vi "Set File Node.vi"(6 "Path":path, 7 "Extension":string, 8 "error in (no error)":errorcluster, 9 "Name":string, 10 "guid":string="3a41ca74-36ec-4aff-9219-9d05c8f91208", 11 "Doc in":refnum<k24>) -> (0 "error out":errorcluster, 3 "Doc out":refnum<k24>)   [LabVIEW 2013, in "Project Wizard.lvlib"]
uses:
  NationalInstruments.VeriStand.SystemStorage
  Project Wizard.lvlib
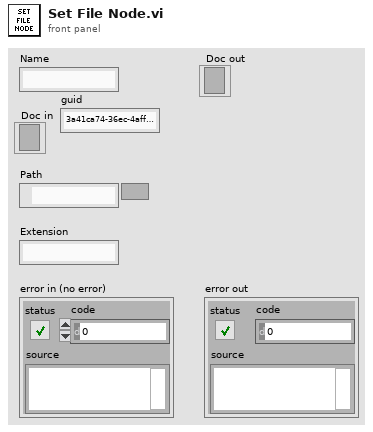
[diagram p1: front panel]
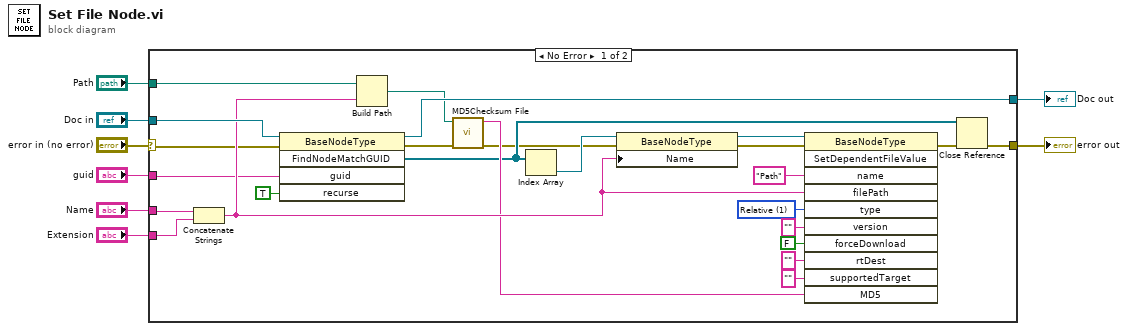
[diagram p0: block diagram]
diagram:
  n1 = case shown="No Error" "error in (no error)" {
    selector: "error in (no error)" -> [w12 w35]
    tunnel: "Doc in" -> [w33 w34]
    tunnel: "Name" -> [w32 _]
    tunnel: "Path" -> [w31 _]
    tunnel: [w29 w34] -> w5
    tunnel: [w28 w35] -> w4
    tunnel: "Extension" -> [w21 _]
    tunnel: "guid" -> [w11 _]
    frame No Error {
      w20 = 1 items=["Absolute", "Relative", "ToCommonDocDir", "ToApplicationDataDir"] ("type")
      n2 = Concatenate Strings(w32, w21) -> (w30:string)
      n3 = invoke class="BaseNodeType" method="FindNodeMatchGUID"(reference=w33, error in=w12, "guid"=w11, "recurse"=TRUE) -> (reference out=w29:refnum<k24>, error out=w10:errorcluster, "FindNodeMatchGUID"=w13:refnum<k24>[])  [unwired: 1 in, 2 out]
      n4 = Build Path(base path=w31, name or relative path=w30) -> (appended path=w27:path)
      n5 = call <vilib>:"MD5Checksum File.vi"("error in (no error)"=w10, "Path"=w27) -> ("error out"=w9:errorcluster, "MD5 message-digest"=w22:string)  [unwired: 8 in]
      n6 = Index Array(array=w13) -> (element=w18:refnum<k24>)  [unwired: 1 in]
      n7 = property class="BaseNodeType"(reference=w18, error in=w9, "Name"=w30) -> (reference out=w17:refnum<k24>, error out=w16:errorcluster)
      n8 = invoke class="BaseNodeType" method="SetDependentFileValue"(reference=w17, error in=w16, "name"="Path", "filePath"=w30, "type"=w20, "version"="", "forceDownload"=FALSE, "rtDest"="", "supportedTarget"="", "MD5"=w22) -> (error out=w14:errorcluster)  [unwired: 1 in, 10 out]
      n9 = Close Reference(reference=w13, error in (no error)=w14) -> (error out=w28:errorcluster)
    }
    frame Error {
    }
  }
  "Doc out" <- w5
  "error out" <- w4
